vi "AES Encrypt (ECB).vi"(7 "Padding":i32(ring)=3 items=["None"=1, "PKCS7"=2, "Zeros"=3, "ANSIX923"=4, "ISO10126"=5], 8 "error in (no error)":errorcluster, 10 "Key":u8[](array[numeric]), 11 "Raw data in":u8[](array[numeric])) -> (0 "error out":errorcluster, 3 "Encrypted data out":u8[](array[numeric]))   [LabVIEW 2021, in "dotNET Crypto Symmetric Encryption.lvlib"]
doc: "Encrypt data using AES using the ECB cipher mode.\n\nA suitable padding mode should be used if the data length does not match a multiple of the block size. The same padding mode must be selected when decrypting the data.\n\nNote - ECB is considered insecure as each identifcal block of data is encrypted into an identical ciphertext block."
uses:
  dotNET Crypto Symmetric Encryption.lvlib
  System.Core
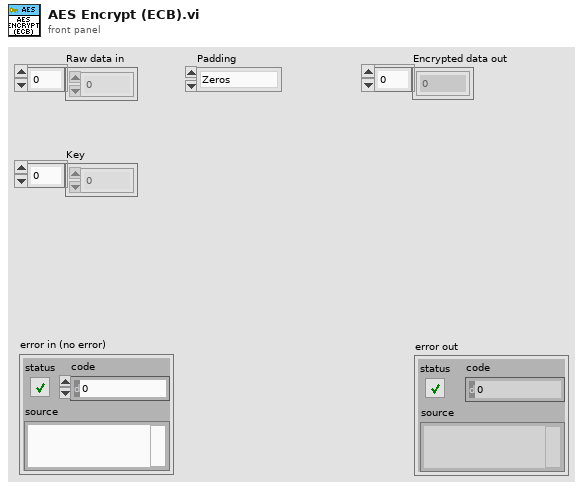
[diagram p1: front panel]
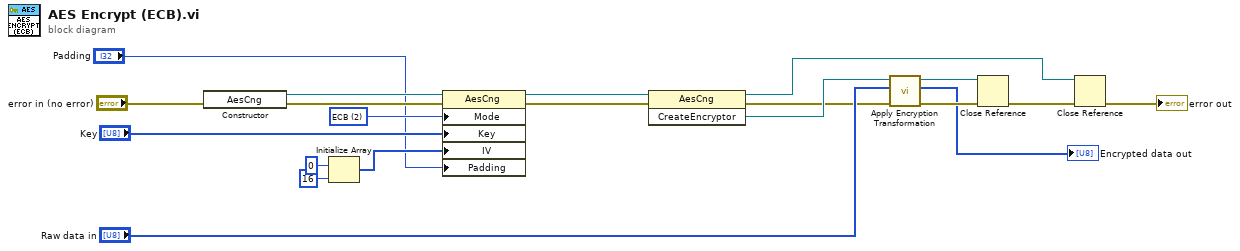
[diagram p0: block diagram]
diagram:
  w18 = 2 items=["CBC"=1, "ECB"=2, "OFB"=3, "CFB"=4, "CTS"=5] ("Mode")
  n1 = constructor class="AesCng"(error in="error in (no error)") -> (reference out=w13:refnum<k24>, error out=w14:errorcluster)  [unwired: 2 in, 1 out]
  n2 = Initialize Array(u8 0, 16 ("dimension size")) -> (w4:u8[])
  n3 = property class="AesCng"(reference=w13, error in=w14, "Mode"=w18, "Key"="Key", "IV"=w4, "Padding"="Padding") -> (reference out=w15:refnum<k24>, error out=w16:errorcluster)
  n4 = invoke class="AesCng" method="CreateEncryptor"(reference=w15, error in=w16) -> (reference out=w9:refnum<k24>, error out=w8:errorcluster, "CreateEncryptor"=w17:refnum<k24>)  [unwired: 1 in]
  n5 = call "Apply Encryption Transformation.vi"("error in (no error)"=w8, "Raw data in"="Raw data in", "CryptoTransform in"=w17) -> ("error out"=w11:errorcluster, "Encrypted data out"=→"Encrypted data out":u8[], "CryptoTransform out"=w6:refnum<k24>)  [unwired: 6 in]
  n6 = Close Reference(reference=w6, error in (no error)=w11) -> (error out=w7:errorcluster)
  n7 = Close Reference(reference=w9, error in (no error)=w7) -> (error out=→"error out":errorcluster)
